vi "TCP Write Entire Buffer.vi"(8 "error in (no error)":errorcluster, 10 "data in":string, 11 "connection ID":refnum<k5>) -> (0 "error out":errorcluster, 2 "bytes written":i32, 3 "connection ID out":refnum<k5>)   [LabVIEW 2014]
doc: "Writes entire buffer to a TCP connection (retrying if a Time Out Error is returned)."
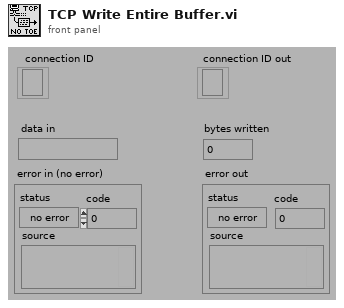
[diagram p1: front panel]
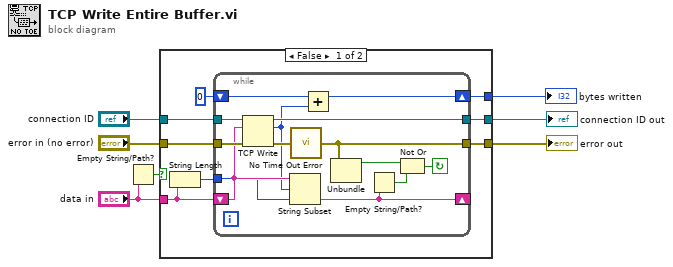
[diagram p0: block diagram]
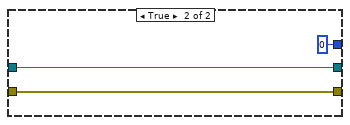
[diagram p2: hidden frame]
diagram:
  n1 = Empty String/Path?(string/path="data in") -> (empty?=w1:bool)
  n2 = case shown="False" w1 {
    tunnel: "data in" -> [w15 _]
    tunnel: [w14 0 ("y")] -> w3
    tunnel: [w12 w32] -> w4
    tunnel: [w10 w31] -> w5
    tunnel: "error in (no error)" -> [w9 w31]
    tunnel: "connection ID" -> [w8 w32]
    frame False {
      n3 = String Length(string=w15) -> (length=w11:i32)
      n4 = while {
        shift-left: 0 ("y") -> [w17]
        shift-right: [w16] -> w14
        tunnel: [w23] -> w12
        tunnel: w11 -> [w25]
        tunnel: [w24] -> w10
        shift-left: w15 -> [w26]
        shift-right: [w22] -> _
        tunnel: w9 -> [w28]
        tunnel: w8 -> [w29]
        stop <- w19 continue-if-true
        n5 = TCP Write(connection ID=w29, data in=w26, error in (no error)=w28) -> (connection ID out=w23:refnum<k5>, bytes written=w18:i32, error out=w27:errorcluster)  [unwired: 1 in]
        n6 = String Subset(string=w26, offset (0)=w18, length (rest)=w25) -> (substring=w22:string)
        n7 = call "No Time Out Error.vi"("error in (no error)"=w27) -> ("error out"=w24:errorcluster)  [unwired: 14 in]
        n8 = Add(x=w17, y=w18) -> (x+y=w16:i32)
        n9 = Unbundle(w24) -> ("status"=w21:bool)  [unwired: 2 out]
        n10 = Empty String/Path?(string/path=w22) -> (empty?=w20:bool)
        n11 = Not Or(1:w20, 2:w21) -> (0:w19:bool)
      }
    }
    frame True {
    }
  }
  "connection ID out" <- w4
  "error out" <- w5
  "bytes written" <- w3
